vi "LBO_cooling.vi"() -> ()   [LabVIEW 2013]
uses:
  <vilib>/Instr/_visa.llb/VISA Configure Serial Port (Instr).vi
  kernel32.dll
panel:
  out "LBO Cooling":bool
  out "LBO Set Temperature":string
  out "LBO Measure Temperature":string="\r\n"
  in  "COMMAND":string="LBOH=0"
  in  "VISA resource name":refnum<visa-resource-name>="COM7"
  out "?":bool
  out "Battery Life":u8(slide)=13 scale=0.0..100.0
  in  "stop":bool
  in  "system_power_status":T1
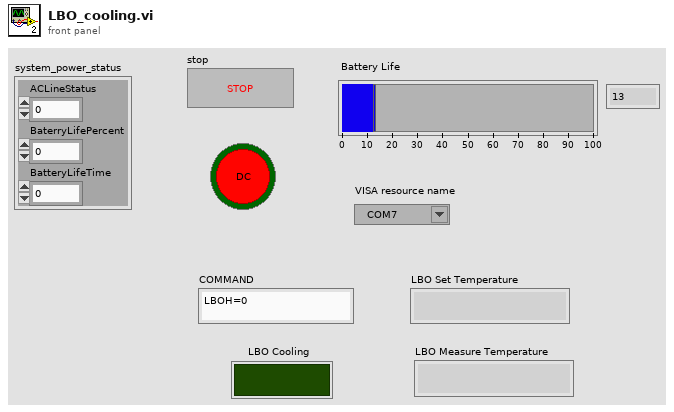
[diagram p1: front panel]
types:
  T1 = cluster{"ACLineStatus":u8, "BaterryLifePercent":u8, "BatteryLifeTime":i32}
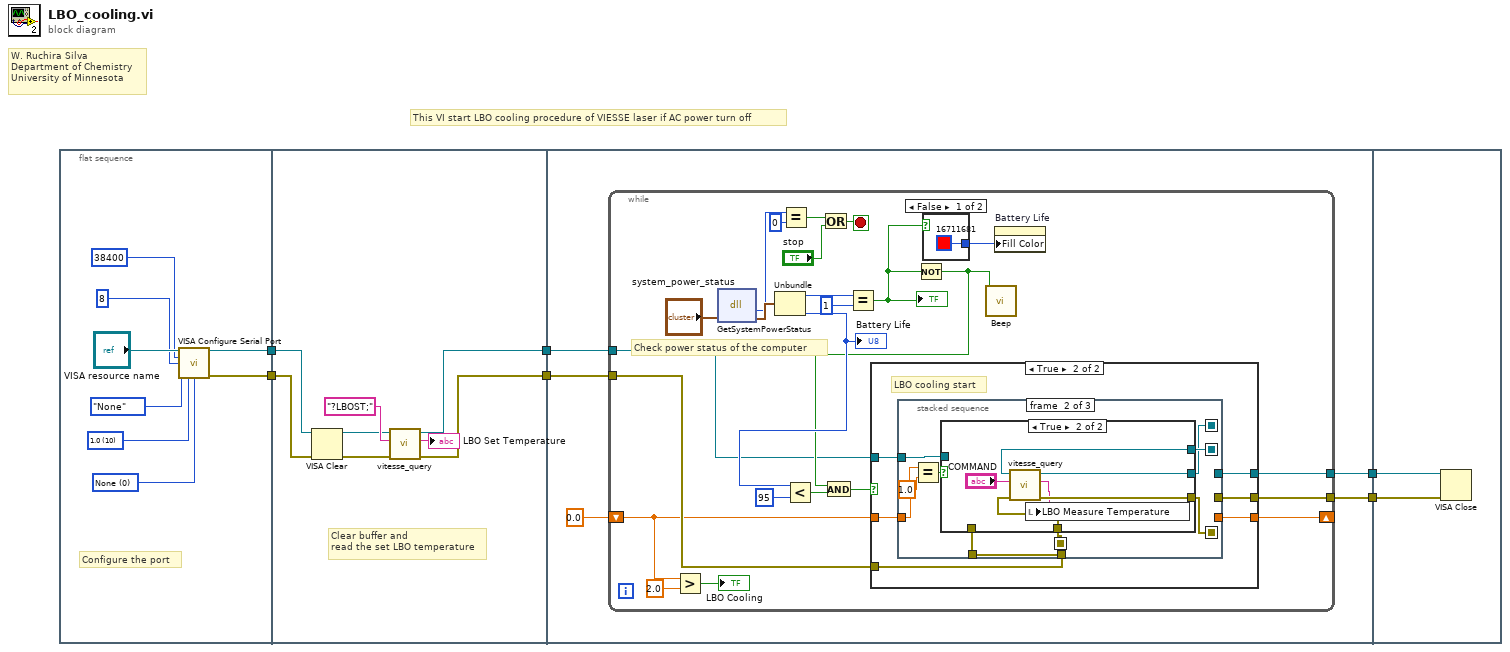
[diagram p0: block diagram]
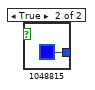
[diagram p2: hidden frame]
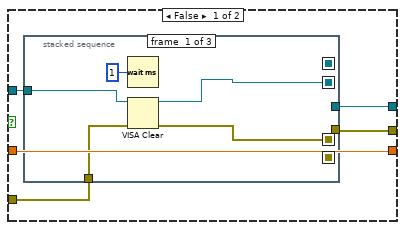
[diagram p3: hidden frame]
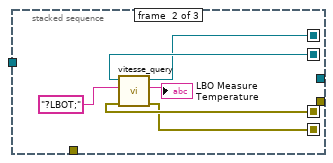
[diagram p4: hidden frame]
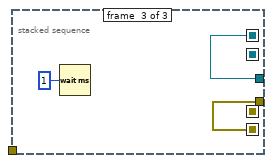
[diagram p5: hidden frame]
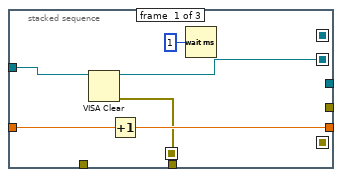
[diagram p6: hidden frame]
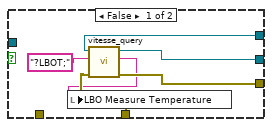
[diagram p7: hidden frame]
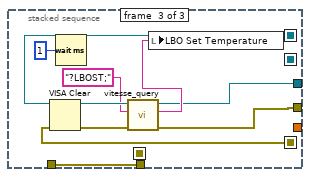
[diagram p8: hidden frame]
diagram:
  # "W. Ruchira Silva\nDepartment of Chemistry\nUniversity of Minnesota"
  # "This VI start LBO cooling procedure of VIESSE laser if AC power turn off"
  n1 = flat-sequence {
    tunnel: [w8] -> w4
    tunnel: [w7] -> w2
    tunnel: w4 -> [w18]
    tunnel: [w21] -> w3
    tunnel: w2 -> [w15]
    tunnel: [w20] -> w1
    tunnel: w3 -> [w27]
    tunnel: w1 -> [w26]
    tunnel: [w25] -> w6
    tunnel: [w24] -> w5
    tunnel: w6 -> [w118]
    tunnel: w5 -> [w117]
    frame #0 {
      w9 = u16 0 items=["None", "XON/XOFF", "RTS/CTS", "XON/XOFF & RTS/CTS", "DTR/DSR", "XON/XOFF & DTR/DSR"] ("flow control (0:none)")
      w10 = u16 10 items=["1.0"=10, "1.5"=15, "2.0"=20] ("stop bits (10: 1 bit)")
      # "Configure the port"
      n2 = call-poly "VISA Configure Serial Port"("VISA resource name"="VISA resource name", "baud rate (9600)"=u32 38400, "data bits (8)"=u16 8, "parity (0:none)"=enum16{"None", "Odd", "Even", "Mark", "Space"}."None", "stop bits (10: 1 bit)"=w10, "flow control (0:none)"=w9) -> ("VISA resource name out"=w8:refnum<visa-resource-name>, "error out"=w7:errorcluster)  [unwired: 8 in]
    }
    frame #1 {
      # "Clear buffer and \nread the set LBO temperature"
      n3 = VISA Clear(VISA resource name=w18, error in (no error)=w15) -> (VISA resource name out=w17:refnum<visa-resource-name>, error out=w16:errorcluster)
      n4 = call "vitesse_query.vi"("error in (no error)"=w16, "write buffer"="?LBOST;", "VISA resource name"=w17) -> ("error out"=w20:errorcluster, "substring"=→"LBO Set Temperature":string, "VISA resource name out"=w21:refnum<visa-resource-name>)  [unwired: 6 in]
    }
    frame #2 {
      n5 = while {
        tunnel: w27 -> [w28]
        tunnel: w26 -> [w44]
        shift-right: [w39] -> _
        shift-left: 0.0 -> [w31]
        tunnel: [w35] -> w25
        tunnel: [w34] -> w24
        stop <- w36 stop-if-true
        # "Check power status of the computer"
        n6 = Greater?(x=w31, y=2.0) -> (0:→"LBO Cooling":bool)
        n7 = dll-call lib="kernel32.dll" fn="GetSystemPowerStatus"("SystemPowerStatus"="system_power_status") -> ("return type"=w49:i32, "SystemPowerStatus"=w51:T1)  [unwired: 3 in, 2 out]
        n8 = Unbundle(w51) -> ("ACLineStatus"=w47:u8, "BatteryLifeTime"=w43:i32)  [unwired: 1 out]
        "Battery Life" <- w43
        n9 = Equal?(x=w49, y=0) -> (x = y?=w38:bool)
        n10 = Less?(x=w43, y=95) -> (x < y?=w40:bool)
        n11 = Or(x=w38, y="stop") -> (x .or. y?=w36:bool)
        n12 = Equal?(x=w47, y=u8 1) -> (x = y?=w33:bool)
        "?" <- w33
        n13 = Not(x=w33) -> (.not. x?=w41:bool)
        n14 = And(x=w41, y=w40) -> (x .and. y?=w42:bool)
        n15 = case shown="True" w42 {
          tunnel: w28 -> [w58 w78]
          tunnel: w44 -> [w57 w77]
          tunnel: w31 -> [w56 w76]
          tunnel: [w56 w75] -> w39
          tunnel: [w55 w74] -> w35
          tunnel: [w54 w73] -> w34
          frame False {
            n16 = stacked-sequence {
              seq-local: [w61 _ _] -> [_ w68 _]
              seq-local: [w60 _ _] -> [_ w67 _]
              seq-local: [_ w65 _] -> [_ _ w70]
              seq-local: [_ w64 _] -> [_ _ w71]
              tunnel: w58 -> [w63 _ _]
              tunnel: w57 -> [w62 _ _]
              tunnel: [_ _ w70] -> w55
              tunnel: [_ _ w71] -> w54
              frame #0 {
                n17 = Wait (ms)(milliseconds to wait=u32 1) -> ()  [unwired: 1 out]
                n18 = VISA Clear(VISA resource name=w63, error in (no error)=w62) -> (VISA resource name out=w61:refnum<visa-resource-name>, error out=w60:errorcluster)
              }
              frame #1 {
                n19 = call "vitesse_query.vi"("error in (no error)"=w67, "write buffer"="?LBOT;", "VISA resource name"=w68) -> ("error out"=w65:errorcluster, "substring"=→"LBO Measure Temperature":string, "VISA resource name out"=w64:refnum<visa-resource-name>)  [unwired: 6 in]
              }
              frame #2 {
                n20 = Wait (ms)(milliseconds to wait=u32 1) -> ()  [unwired: 1 out]
              }
            }
          }
          frame True {
            # "LBO cooling start"
            n21 = stacked-sequence {
              seq-local: [w80 _ _] -> [_ w88 _]
              seq-local: [w79 _ _] -> [_ w89 _]
              seq-local: [_ w87 _] -> [_ _ w109]
              seq-local: [_ w86 _] -> [_ _ w110]
              tunnel: w78 -> [w82 w94 _]
              tunnel: w77 -> [w81 w93 w115]
              tunnel: w76 -> [w84 w91 _]
              tunnel: [w83 _ _] -> w75
              tunnel: [_ _ w115] -> _
              tunnel: [_ _ w108] -> w74
              tunnel: [_ _ w107] -> w73
              frame #0 {
                n22 = VISA Clear(VISA resource name=w82, error in (no error)=w81) -> (VISA resource name out=w79:refnum<visa-resource-name>, error out=w80:errorcluster)
                n23 = Increment(x=w84) -> (x+1=w83:dbl)
                n24 = Wait (ms)(milliseconds to wait=u32 1) -> ()  [unwired: 1 out]
              }
              frame #1 {
                n25 = Equal?(x=w91, y=1.0) -> (x = y?=w92:bool)
                n26 = case shown="True" w92 {
                  tunnel: w94 -> [_ _]
                  tunnel: w93 -> [_ _]
                  tunnel: [w96 w105] -> w87
                  tunnel: [w98 w104] -> w86
                  tunnel: w89 -> [w99 w103]
                  tunnel: w88 -> [w97 w102]
                  frame False {
                    n27 = call "vitesse_query.vi"("error in (no error)"=w97, "write buffer"="?LBOT;", "VISA resource name"=w99) -> ("error out"=w96:errorcluster, "substring"=w95:string, "VISA resource name out"=w98:refnum<visa-resource-name>)  [unwired: 6 in]
                    n28 = local write "LBO Measure Temperature"(w95) -> ()
                  }
                  frame True {
                    n29 = call "vitesse_query.vi"("error in (no error)"=w102, "write buffer"="COMMAND", "VISA resource name"=w103) -> ("error out"=w105:errorcluster, "substring"=w101:string, "VISA resource name out"=w104:refnum<visa-resource-name>)  [unwired: 6 in]
                    n30 = local write "LBO Measure Temperature"(w101) -> ()
                  }
                }
              }
              frame #2 {
                n31 = VISA Clear(VISA resource name=w110, error in (no error)=w109) -> (VISA resource name out=w114:refnum<visa-resource-name>, error out=w113:errorcluster)
                n32 = Wait (ms)(milliseconds to wait=u32 1) -> ()  [unwired: 1 out]
                n33 = call "vitesse_query.vi"("error in (no error)"=w113, "write buffer"="?LBOST;", "VISA resource name"=w114) -> ("error out"=w108:errorcluster, "substring"=w111:string, "VISA resource name out"=w107:refnum<visa-resource-name>)  [unwired: 6 in]
                n34 = local write "LBO Set Temperature"(w111) -> ()
              }
            }
          }
        }
        n35 = case shown="False" w33 {
          tunnel: [u32 16711681 u32 1048815] -> w32
          frame False {
          }
          frame True {
          }
        }
        n36 = call <vilib>:"Beep.vi"("use system alert? (T)"=w41) -> ()  [unwired: 11 in]
        n37 = property on="Battery Life" class="Slide (strict)"("Fill Color"=w32) -> ()  [unwired: 2 in, 2 out]
      }
    }
    frame #3 {
      n38 = VISA Close(VISA resource name=w117, error in (no error)=w118) -> ()  [unwired: 1 out]
    }
  }
